vi "Read configured channels.vi"(8 "error in (no error)":errorcluster, 11 "fixed channel tag bus module configuration in":refnum<class "fixed channel tag bus module configuration.lvclass">) -> (0 "error out":errorcluster, 2 "configured channels":refnum<class "TBM channel.lvclass">[](array[class]), 3 "fixed channel tag bus module configuration out":refnum<class "fixed channel tag bus module configuration.lvclass">)   [LabVIEW 2013]
uses:
  fixed channel tag bus module configuration.lvclass
  <vilib>/NI/Tag Bus Module Framework/channel/TBM channel.lvclass
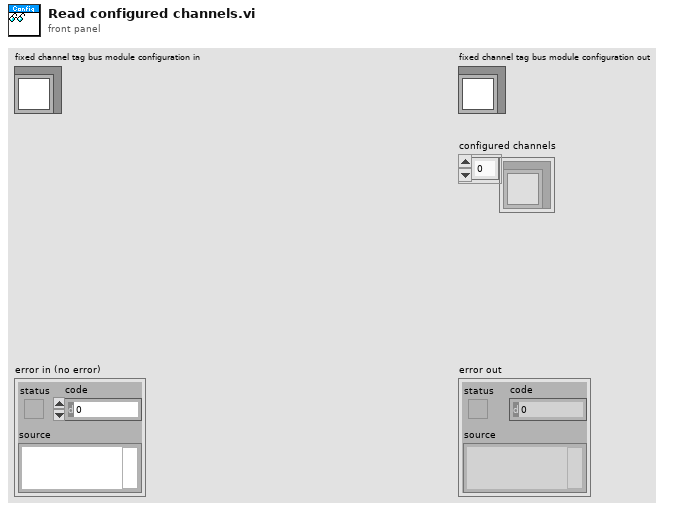
[diagram p1: front panel]
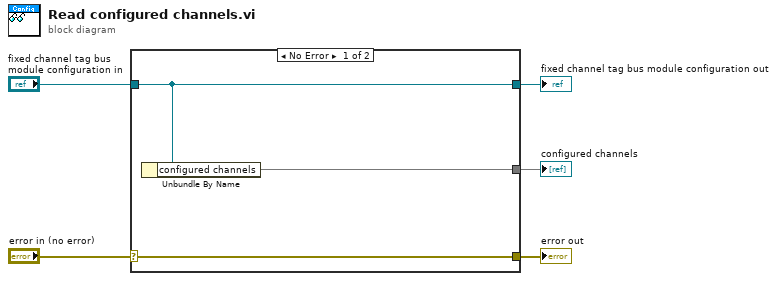
[diagram p0: block diagram]
diagram:
  n1 = case shown="No Error" "error in (no error)" {
    selector: "error in (no error)" -> [w8 w9]
    tunnel: [w8 w9] -> w4
    tunnel: [w7 w10] -> w2
    tunnel: "fixed channel tag bus module configuration in" -> [w7 w10]
    tunnel: [w6 _] -> w1
    frame No Error {
      n2 = Unbundle By Name(w7) -> ("configured channels"=w6)
    }
    frame Error {
    }
  }
  "error out" <- w4
  "fixed channel tag bus module configuration out" <- w2
  "configured channels" <- w1
